vi "haskel graph.vi"() -> ()   [LabVIEW 2019]
uses:
  <vilib>/Analysis/NI_AALPro.lvlib
panel:
  out "residue":dbl
  out "-x":dbl
  out "B":dbl
  out "A":dbl
  out "XY Graph":cluster{dbl[], dbl[]}[](graph)
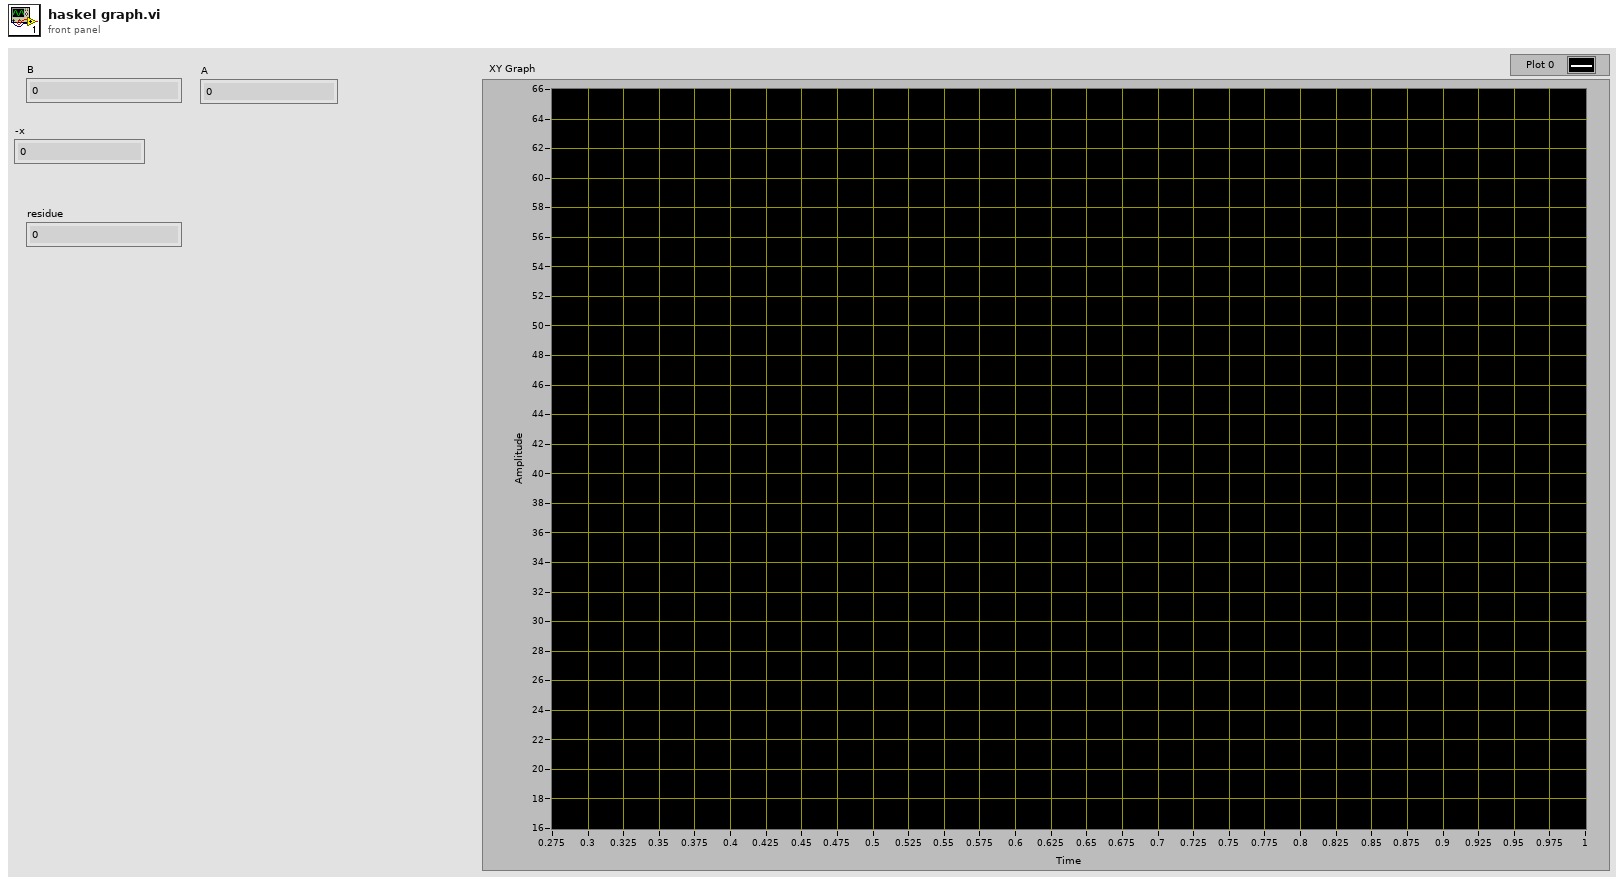
[diagram p1: front panel]
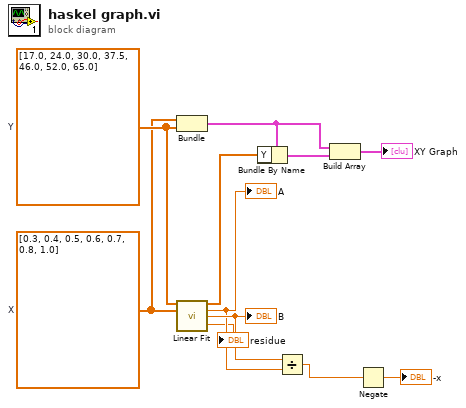
[diagram p0: block diagram]
diagram:
  w11 = dbl[] [17.0, 24.0, 30.0, 37.5, 46.0, 52.0, 65.0]  # Y
  w10 = dbl[] [0.3, 0.4, 0.5, 0.6, 0.7, 0.8, 1.0]  # X
  n1 = Bundle("X"=w10, "Y"=w11) -> (w8:cluster{"X":dbl[], "Y":dbl[]})  [unwired: 1 in]
  n2 = call <vilib>:"Linear Fit.vi"("Y"=w11, "X"=w10) -> ("Best Linear Fit"=w7:dbl[], "slope"=w4:dbl, "intercept"=w5:dbl, "residue"=→"residue":dbl)  [unwired: 9 in, 1 out]
  "A" <- w4
  "B" <- w5
  n3 = Bundle By Name(cluster=w8, "Y"=w7) -> (w6:cluster{"X":dbl[], "Y":dbl[]})
  n4 = Divide(x=w5, y=w4) -> (x/y=w3:dbl)
  n5 = Build Array(w8, w6) -> (→"XY Graph":cluster{"X":dbl[], "Y":dbl[]}[])
  n6 = Negate(x=w3) -> (-x=→"-x":dbl)
